vi "Rotate.vi"(8 "error in (no error)":errorcluster, 10 "Rotation Angle (Deg.)":dbl, 11 "Angle in":refnum<class "Angle.lvclass">) -> (0 "error out":errorcluster, 2 "New Angle":dbl, 3 "Angle out":refnum<class "Angle.lvclass">)   [LabVIEW 2011, in "Angle.lvclass"]
doc: "Calculates a new angle that is the old angle rotated by the rotation angle."
uses:
  Angle.lvclass
  Angle.lvclass/Angle.ctl
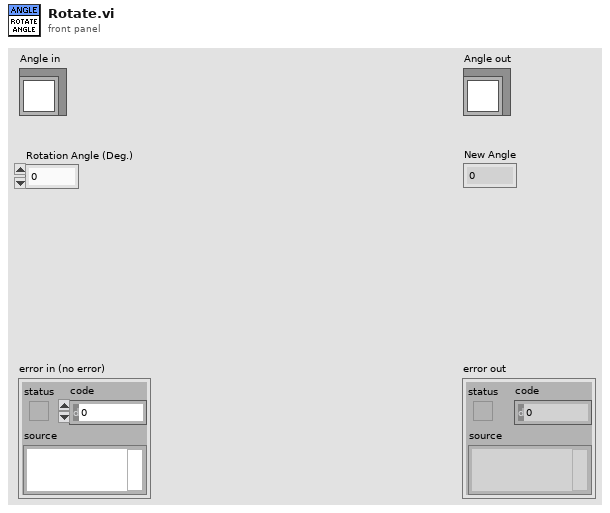
[diagram p1: front panel]
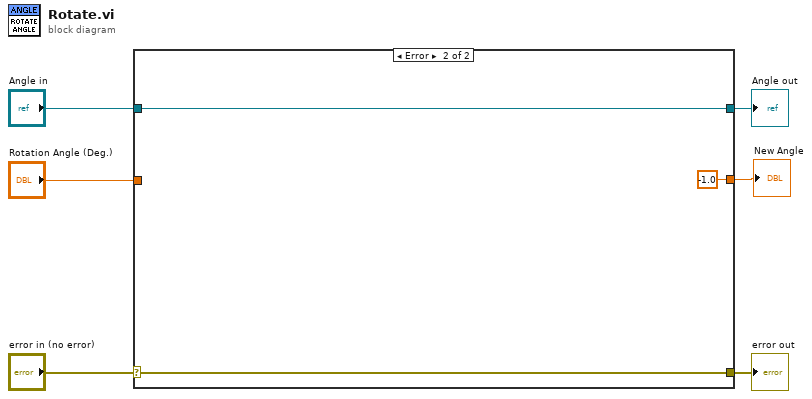
[diagram p0: block diagram]
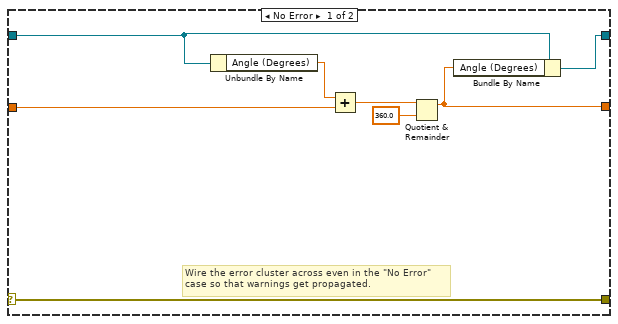
[diagram p2: hidden frame]
diagram:
  n1 = case shown="Error" "error in (no error)" {
    selector: "error in (no error)" -> [w14 w17]
    tunnel: [w14 w17] -> w5
    tunnel: [w8 w16] -> w3
    tunnel: "Angle in" -> [w9 w16]
    tunnel: "Rotation Angle (Deg.)" -> [w12 _]
    tunnel: [w7 -1.0] -> w1
    frame No Error {
      # "Wire the error cluster across even in the \"No Error\"\ncase so that warnings get propagated."
      n2 = Unbundle By Name(w9) -> ("Angle (Degrees)"=w13:dbl)
      n3 = Add(x=w13, y=w12) -> (x+y=w11:dbl)
      n4 = Quotient & Remainder(x=w11, y=360.0) -> (x-y*floor(x/y)=w7:dbl)  [unwired: 1 out]
      n5 = Bundle By Name(cluster=w9, "Angle (Degrees)"=w7) -> (w8:refnum<class "Angle.lvclass">)
    }
    frame Error {
    }
  }
  "error out" <- w5
  "Angle out" <- w3
  "New Angle" <- w1
